vi "scanner delete.vi"(8 "error in":errorcluster, 10 "Index":i32, 11 "Config.Scanners":string[](array[string])) -> (0 "error out":errorcluster, 1 "Valid":bool, 2 "Error":string, 3 "Config.Scanners":string[](array[string]))   [LabVIEW 2023, in "User Interface.lvlib"]
uses:
  User Interface.lvlib
panel:
  # "Output Indicators"
  # "Input Controls"
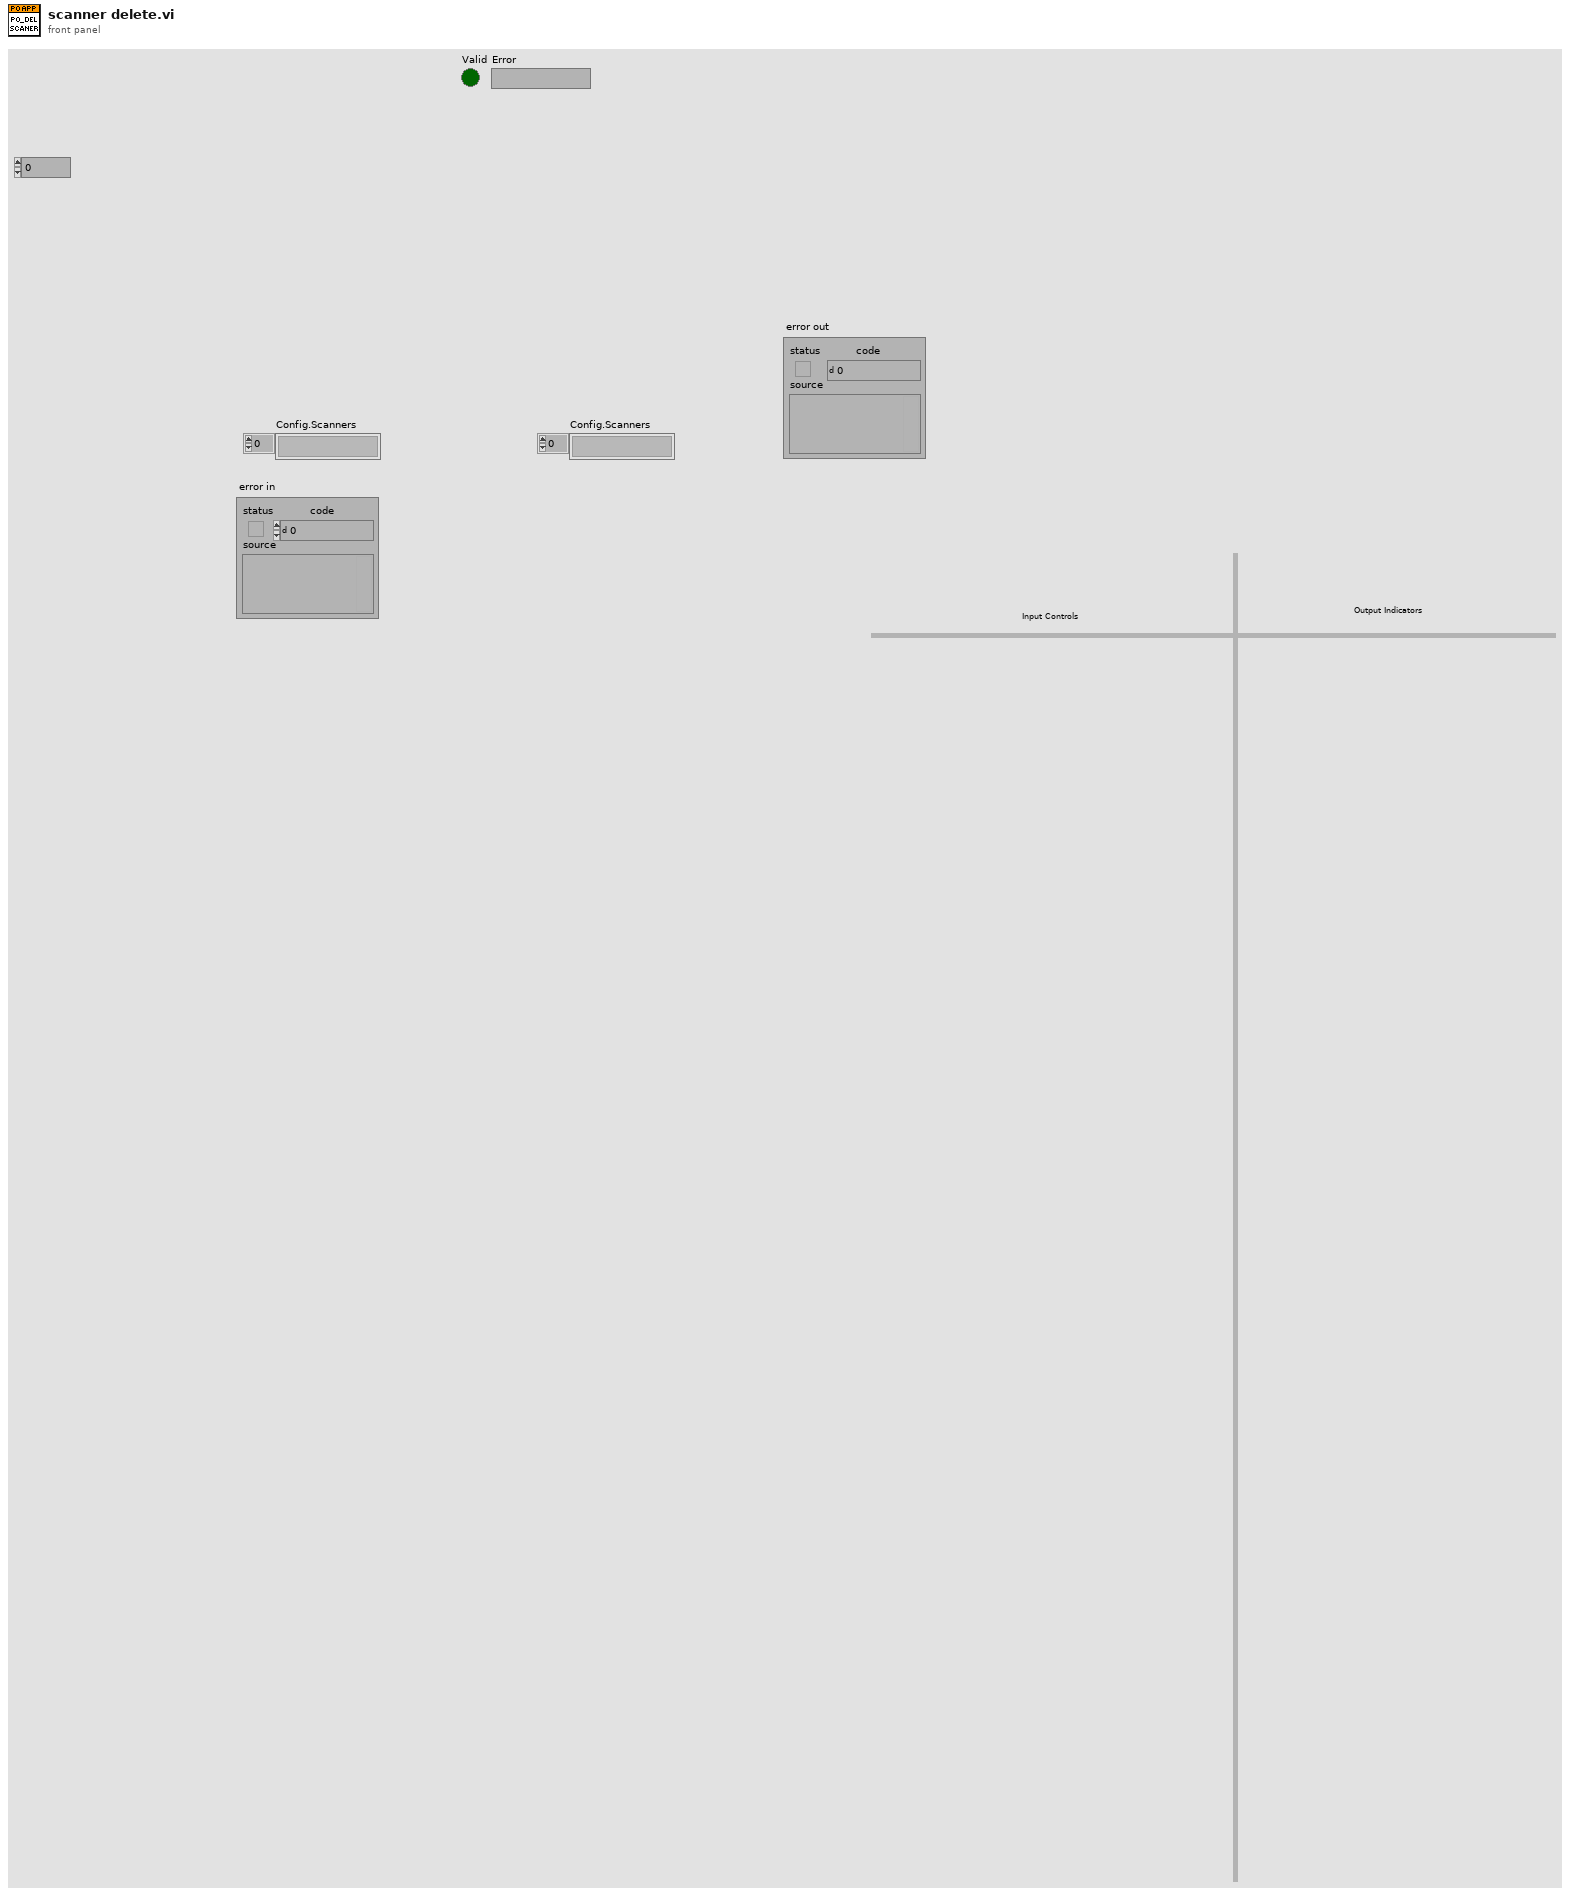
[diagram p1: front panel]
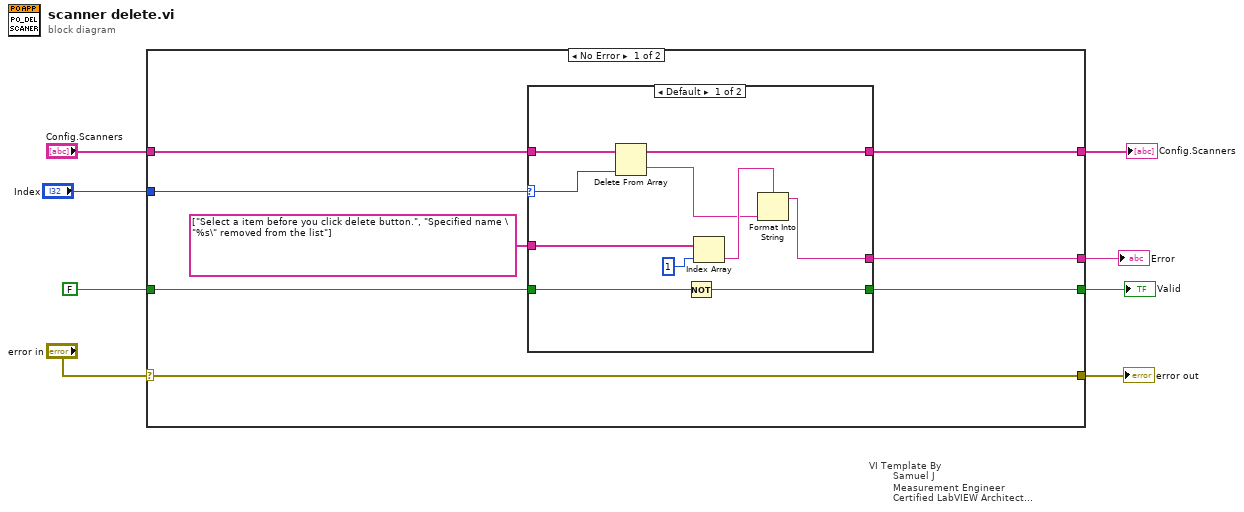
[diagram p0: block diagram]
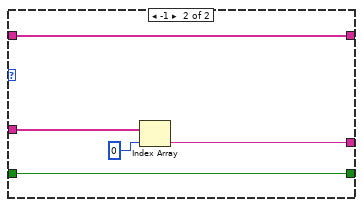
[diagram p2: hidden frame]
diagram:
  n1 = case "VI Template By\n        Samuel J\n        Measurement Engineer\n        Certified LabVIEW Architect\n        Vestas Technology R&D Chennai" shown="No Error" "error in" {
    selector: "error in" -> [w16 w34]
    tunnel: [w16 w34] -> w7
    tunnel: [w12 w33] -> w5
    tunnel: "Config.Scanners" -> [w13 w33]
    tunnel: [w15 w32] -> w3
    tunnel: FALSE -> [w14 w32]
    tunnel: [w10 _] -> w2
    tunnel: "Index" -> [w9 _]
    frame No Error {
      n2 = case shown="Default" w9 {
        selector: w9 -> [w19 _]
        tunnel: w13 -> [w20 w31]
        tunnel: [w18 w31] -> w12
        tunnel: [w26 w30] -> w15
        tunnel: w14 -> [w25 w30]
        tunnel: string[] ["Select a item before you click delete button.", "Specified name \"%s\" removed from the list"] -> [w24 w28]
        tunnel: [w23 w27] -> w10
        frame Default {
          n3 = Delete From Array(array=w20, index=w19) -> (deleted portion=w17:string, array with subset deleted=w18:string[])  [unwired: 1 in]
          n4 = Not(x=w25) -> (.not. x?=w26:bool)
          n5 = Index Array(array=w24, index=1) -> (element=w21:string)
          n6 = Format Into String(format string=w21, w17) -> (resulting string=w23:string)  [unwired: 2 in, 1 out]
        }
        frame -1 {
          n7 = Index Array(array=w28, index=0) -> (element=w27:string)
        }
      }
    }
    frame Error {
    }
  }
  "error out" <- w7
  "Config.Scanners" <- w5
  "Valid" <- w3
  "Error" <- w2
